vi "Fc_to_read_TCP.vi"(11 "path_mainmenu":path) -> (1 "Hhostname":string, 2 "Timeout ms":i32, 3 "Port":i32)   [LabVIEW 2022 SP3]
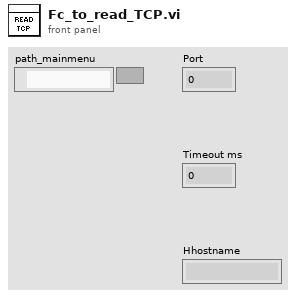
[diagram p1: front panel]
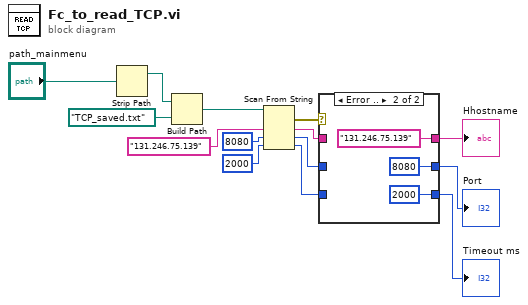
[diagram p0: block diagram]
diagram:
  n1 = Strip Path(path="path_mainmenu") -> (stripped path=w3:path)  [unwired: 1 out]
  n2 = Build Path(base path=w3, name or relative path=path "TCP_saved.txt" ("default name")) -> (appended path=w4:path)
  n3 = Scan From String(w4, default 1="131.246.75.139" ("hostname"), default 2=8080, default 3=2000 ("timeout ms")) -> (w8:errorcluster, output 1=w12:string, output 2=w13:i32, output 3=w14:i32)  [unwired: 2 in, 1 out]
  n4 = case shown="Error .." w8 {
    tunnel: [w17 "131.246.75.139" ("hostname")] -> w9
    tunnel: [w16 8080] -> w10
    tunnel: [w15 2000 ("timeout ms")] -> w11
    tunnel: w12 -> [w17 _]
    tunnel: w13 -> [w16 _]
    tunnel: w14 -> [w15 _]
    frame No Error {
    }
    frame Error {
    }
  }
  "Timeout ms" <- w11
  "Port" <- w10
  "Hhostname" <- w9
